vi "StartService.vi"(8 "error in (no error)":errorcluster, 9 "Args":string, 10 "Executable":string, 11 "Service Name":string) -> (0 "error out":errorcluster)   [LabVIEW 2019, in "MicronManager.lvclass"]
uses:
  MicronManager.lvclass
  <vilib>/SLL Toolkit/SLL Debug/SLL Debug.lvlib
  <vilib>/SLL Toolkit/SLL File IO/SLL File IO.lvlib
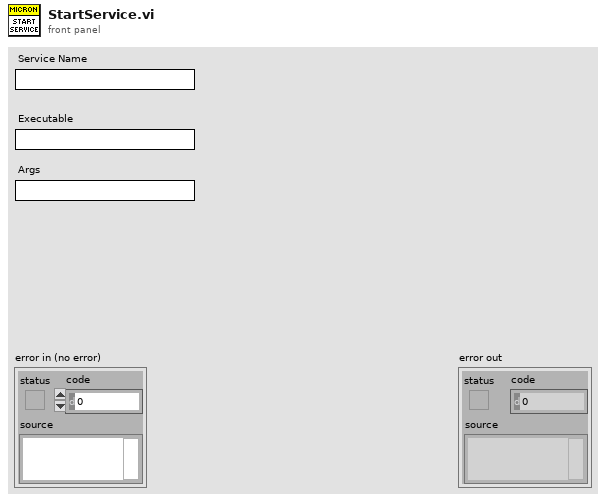
[diagram p1: front panel]
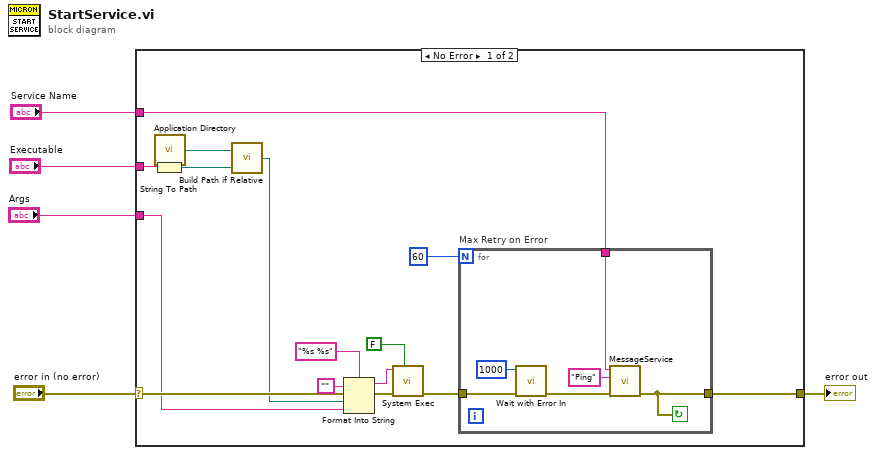
[diagram p0: block diagram]
diagram:
  n1 = case shown="No Error" "error in (no error)" {
    selector: "error in (no error)" -> [w19 w27]
    tunnel: [w17 w27] -> w4
    tunnel: "Executable" -> [w9 _]
    tunnel: "Service Name" -> [w16 _]
    tunnel: "Args" -> [w12 _]
    frame No Error {
      n2 = String To Path(string=w9) -> (path=w8:path)
      n3 = call <vilib>:"Application Directory.vi"() -> ("Application Directory"=w7:path)
      n4 = call <vilib>:"Build Path if Relative.vi"("Relative or Absolute Path"=w8, "Base Path"=w7) -> ("Path Out"=w6:path)
      n5 = Format Into String(format string="%s %s", initial string="", error in=w19, w6, w12) -> (resulting string=w10:string, error out=w14:errorcluster)
      n6 = call <vilib>:"System Exec.vi"("wait until completion? (T)"=FALSE, "error in (no error)"=w14, "command line"=w10) -> ("error out"=w18:errorcluster)  [unwired: 5 in, 3 out]
      n7 = for "Max Retry on Error" {
        N: 60 -> [_]
        tunnel: w16 -> [w25]
        tunnel: w18 -> [w26]
        tunnel: [w23] -> w17
        stop <- w23 continue-if-true
        n8 = call <vilib>:"Wait with Error In.vi"("error in (no error)"=w26, "milliseconds to wait"=u32 1000) -> ("error out"=w22:errorcluster)  [unwired: 9 in]
        n9 = call "MessageService.vi"("error in (no error)"=w22, "Message"="Ping", "Service Name"=w25) -> ("error out"=w23:errorcluster)  [unwired: 7 in, 1 out]
      }
    }
    frame Error {
    }
  }
  "error out" <- w4
